vi "Flatness SLM.vi"(2 "Action":u16(ring) items=["Read", "Initialize"]) -> (8 "flatness":dbl[][](array[numeric]))   [LabVIEW 2014]
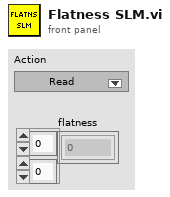
[diagram p1: front panel]
types:
  T1 = typedef "IMAQ Image.ctl" = refnum<image>
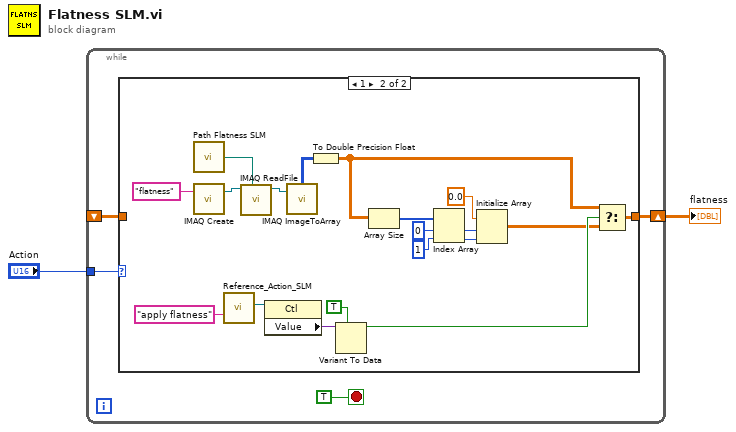
[diagram p0: block diagram]
diagram:
  n1 = while {
    shift-right: [w3] -> w1
    shift-left: _ -> [w4]
    tunnel: "Action" -> [w5]
    stop <- TRUE stop-if-true
    n2 = case shown="1" w5 {
      tunnel: w4 -> [w7 _]
      tunnel: [w7 w17] -> w3
      frame 0, Default {
      }
      frame 1 {
        n3 = call "Path Flatness SLM.vi"() -> ("flatness path"=w24:path)  [unwired: 15 in]
        n4 = call "IMAQ Create"("Image Name"="flatness") -> ("New Image"=w26:T1)  [unwired: 3 in, 2 out]
        n5 = call "Reference_Action_SLM.vi"("Control Name"="apply flatness") -> ("Ref OUT"=w20:refnum<vi>)  [unwired: 12 in, 2 out]
        n6 = call "IMAQ ReadFile"("File Path"=w24, "Image"=w26) -> ("Image Out"=w25:T1)  [unwired: 3 in, 6 out]
        n7 = property class="Ctl"(reference=w20) -> ("Value"=w21:variant)  [unwired: 1 in, 2 out]
        n8 = call "IMAQ ImageToArray"("Image"=w25) -> ("Image Pixels (U8)"=w22:u8[][])  [unwired: 2 in, 5 out]
        n9 = To Double Precision Float(number=w22) -> (double precision float=w15:dbl[][])
        n10 = Variant To Data(type=TRUE, Variant=w21) -> (data=w16:bool)  [unwired: 1 in, 1 out]
        n11 = Array Size(array=w15) -> (size(s)=w13:i32[])
        n12 = Index Array(array=w13, index #1=0 ("index"), index #2=1 ("index")) -> (element #1=w11:i32, element #2=w10:i32)
        n13 = Initialize Array(0.0 ("element"), w11, w10) -> (w8:dbl[][])
        n14 = Select(t=w15, s=w16, f=w8) -> (s? t:f=w17:dbl[][])
      }
    }
  }
  "flatness" <- w1
